vi "ReadIni.vi"(8 "Error In":errorcluster) -> (0 "Error Out":errorcluster, 3 "InternalData":T1)   [LabVIEW 2017, in "Client.lvlib" / "CommsFrameWork.lvlib"]
uses:
  CommsFrameWork.lvlib
  TypeDefs/InternalData.ctl
  ClientGlobals.vi
  <vilib>/Utility/config.llb/Read Key (String).vi
  <vilib>/Utility/config.llb/NI_LVConfig.lvlib
  Client.lvlib
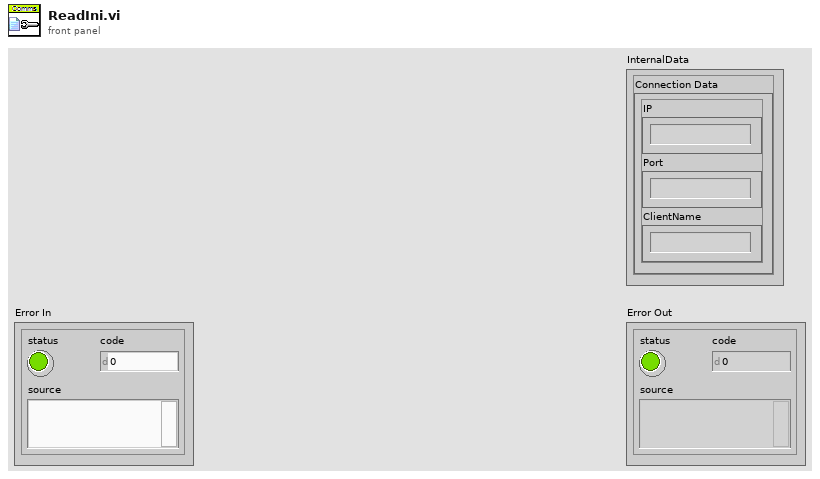
[diagram p1: front panel]
types:
  T1 = typedef "Client.lvlib/CommsFrameWork.lvlib/InternalData.ctl" = cluster{"Connection Data":cluster{"IP":string, "Port":string, "ClientName":string}}
  T2 = typedef "NI_LVConfig.lvlib/Config Data RefNum.ctl" = refnum<k1>
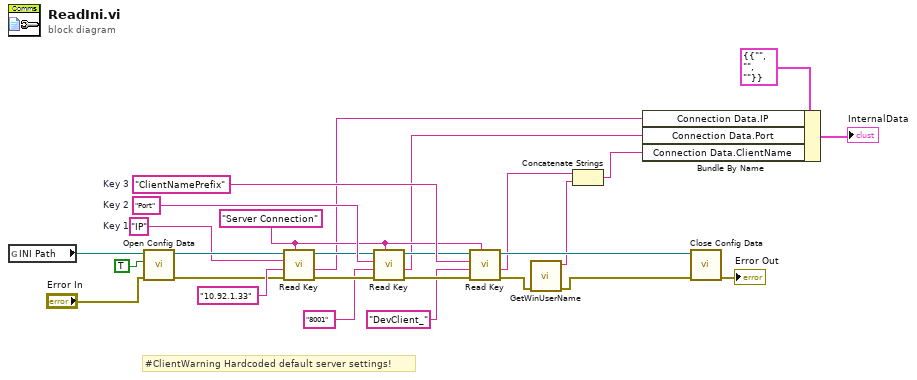
[diagram p0: block diagram]
diagram:
  w22 = "ClientNamePrefix"  # Key 3
  w21 = "Port"  # Key 2
  w20 = "IP"  # Key 1
  w19 = "Server Connection" ("section")
  # "#ClientWarning Hardcoded default server settings!"
  n1 = global read "ClientGlobals.vi" "INI Path"() -> (w1:path)
  n2 = call <vilib>:"Open Config Data.vi"("error in (no error)"="Error In", "create file if necessary (T)"=TRUE ("create file if necessary? (T)"), "configuration file path"=w1) -> ("error out"=w23:errorcluster, "refnum"=w24:T2)  [unwired: 6 in, 1 out]
  n3 = call-poly <vilib>:"Read Key.vi"("section"=w19, "error in (no error)"=w23, "default value"="10.92.1.33", "key"=w20, "refnum"=w24) -> ("error out"=w15:errorcluster, "value"=w13:string, "refnum out"=w16:T2)  [unwired: 1 in, 3 out]
  n4 = call-poly <vilib>:"Read Key.vi"("section"=w19, "error in (no error)"=w15, "default value"="8001", "key"=w21, "refnum"=w16) -> ("error out"=w18:errorcluster, "value"=w12:string, "refnum out"=w17:T2)  [unwired: 1 in, 3 out]
  n5 = call-poly <vilib>:"Read Key.vi"("section"=w19, "error in (no error)"=w18, "default value"="DevClient_", "key"=w22, "refnum"=w17) -> ("error out"=w5:errorcluster, "value"=w6:string, "refnum out"=w26:T2)  [unwired: 1 in, 3 out]
  n6 = call "GetWinUserName.vi"("Error In"=w5) -> ("Error Out"=w4:errorcluster, "Windows User Name"=w8:string)  [unwired: 9 in]
  n7 = Concatenate Strings(w6, w8) -> (w7:string)
  n8 = Bundle By Name(cluster=T1 {"Connection Data"={"IP"="", "Port"="", "ClientName"=""}} ("InternalData"), "Connection Data.IP"=w13, "Connection Data.Port"=w12, "Connection Data.ClientName"=w7) -> (→"InternalData":T1)
  n9 = call <vilib>:"Close Config Data.vi"("error in (no error)"=w4, "refnum"=w26) -> ("error out"=→"Error Out":errorcluster)  [unwired: 1 in, 8 out]
